vi "Send Launch Subscriber.vi"(7 "Message Priority (Normal)":T1=enum."Normal", 8 "error in (no error)":errorcluster, 10 "Actor to Launch":refnum<class "Actor.lvclass">, 11 "Actor in":refnum<class "Actor.lvclass">) -> (0 "error out":errorcluster, 1 "Dropped?":bool, 3 "Actor out":refnum<class "Actor.lvclass">)   [LabVIEW 2020, in "Publisher.lvlib" / "Launch Subscriber Msg.lvclass"]
doc: "This VI sends the message to an actor."
uses:
  Launch Subscriber Msg.lvclass
  PPL/HDH.Actor Framework.Core.Actor.lvlibp/1abvi3w/vi.lib/ActorFramework/Actor/Actor.lvclass
  PPL/HDH.Actor Framework.Core.Actor.lvlibp/1abvi3w/vi.lib/ActorFramework/Message Enqueuer/Message Priority.ctl
  C:/Current projects/WS/Framework/Framework/Actors/Publisher/Publisher Messages/Publisher Msg/Publisher Msg.lvclass
  Launch Subscriber Msg.lvclass/Launch Subscriber Msg.ctl
  Publisher Msg/Publisher Msg.lvclass
  PPL/HDH.Actor Framework.Core.Actor.lvlibp/1abvi3w/vi.lib/ActorFramework/Message Enqueuer/Message Enqueuer.lvclass
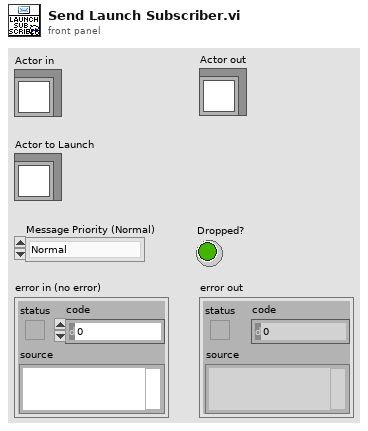
[diagram p1: front panel]
types:
  T1 = typedef "HDH.Actor Framework.Core.Actor.lvlibp/Message Enqueuer.lvclass/Message Priority.ctl" = enum16{"Low", "Normal", "High"}
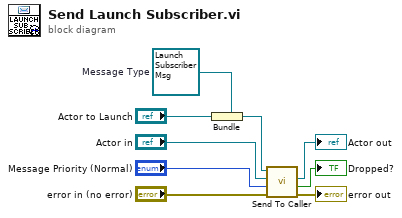
[diagram p0: block diagram]
diagram:
  w9 = refnum<class "Launch Subscriber Msg.lvclass"> refnum  # Message Type
  n1 = Bundle(cluster=w9, "Actor to Launch") -> (w7:refnum<class "Launch Subscriber Msg.lvclass">)
  n2 = call "Send To Caller.vi"("error in (no error)"="error in (no error)", "Message Priority (Normal)"="Message Priority (Normal)", "Actor in"="Actor in", "Publisher Msg in"=w7) -> ("error out"=→"error out":errorcluster, "Msg Dropped?"=→"Dropped?":bool, "Actor out"=→"Actor out":refnum<class "Actor.lvclass">)  [unwired: 5 in]
